vi "Get Pulse State.vi"(8 "error in (no error)":errorcluster, 11 "Red Pitaya Digitizer in":refnum<class "Red Pitaya Digitizer.lvclass">) -> (0 "error out":errorcluster, 1 "Data ready":bool, 2 "Armed":bool, 3 "Red Pitaya Digitizer out":refnum<class "Red Pitaya Digitizer.lvclass">, 4 "Recording compleste":bool)   [LabVIEW 2021, in "Red Pitaya Digitizer.lvclass"]
uses:
  Red Pitaya Digitizer.lvclass
  Red Pitaya Digitizer.lvclass/Red Pitaya Digitizer.ctl
  Read RP Instrument.vi
  Write RP Instrument.vi
  RP Core/RP Instrument/RP Instrument.lvclass
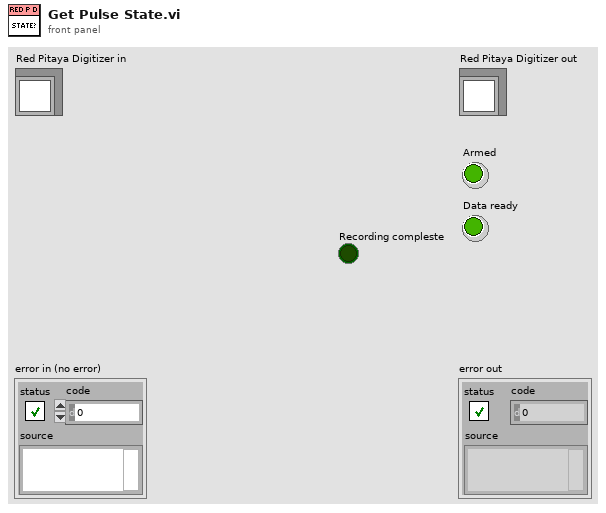
[diagram p1: front panel]
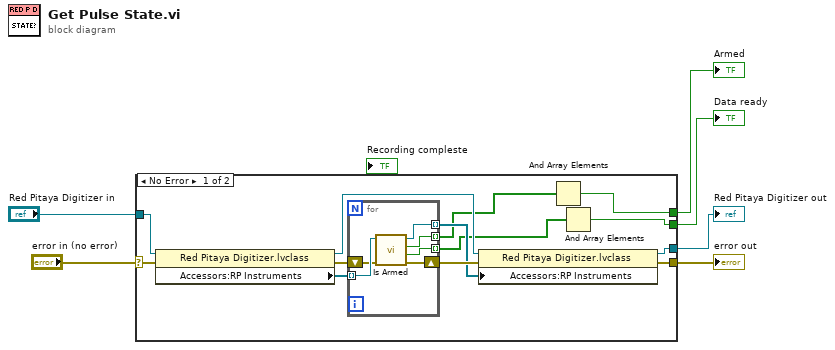
[diagram p0: block diagram]
diagram:
  n1 = case shown="No Error" "error in (no error)" {
    selector: "error in (no error)" -> [w16 w27]
    tunnel: "Red Pitaya Digitizer in" -> [w19 w26]
    tunnel: [w12 w26] -> w4
    tunnel: [w11 w27] -> w3
    tunnel: [w9 _] -> w2
    tunnel: [w7 _] -> w1
    frame No Error {
      n2 = property class="Red Pitaya Digitizer.lvclass"(reference=w19, error in=w16) -> (reference out=w15:refnum<class "Red Pitaya Digitizer.lvclass">, error out=w17:errorcluster, "Accessors:RP Instruments"=w18:refnum<class "RP Instrument.lvclass">[])
      n3 = for {
        tunnel: w18 -> [w25] mode=indexing
        tunnel: [w22] -> w13 mode=indexing
        tunnel: [w21] -> w10 mode=indexing
        tunnel: [w20] -> w8 mode=indexing
        shift-right: [w23] -> w14
        shift-left: w17 -> [w24]
        n4 = call-dynamic "Is Armed.vi"("error in (no error)"=w24, "RP Instrument in"=w25) -> ("error out"=w23:errorcluster, "Finished"=w20:bool, "Armed"=w21:bool, "RP Instrument out"=w22:refnum<class "RP Instrument.lvclass">)  [unwired: 5 in, 1 out]
      }
      n5 = property class="Red Pitaya Digitizer.lvclass"(reference=w15, error in=w14, "Accessors:RP Instruments"=w13) -> (reference out=w12:refnum<class "Red Pitaya Digitizer.lvclass">, error out=w11:errorcluster)
      n6 = And Array Elements(Boolean array=w10) -> (logical AND=w9:bool)
      n7 = And Array Elements(Boolean array=w8) -> (logical AND=w7:bool)
    }
    frame Error {
    }
  }
  "error out" <- w3
  "Red Pitaya Digitizer out" <- w4
  "Armed" <- w2
  "Data ready" <- w1
